vi "visualisation.vi"(8 "Joint B":dbl(knob)=5.611498737356196 scale format="%#.1f", 9 "Joint A":dbl(knob)=5.611498737356196 scale format="%#.1f", 10 "Length B":dbl(slide)=35.714285714285715 scale=10.0..80.0, 11 "Length A":dbl(slide)=70.71428571428572 scale=10.0..80.0) -> (3 "Picture":picture)   [LabVIEW 2016]
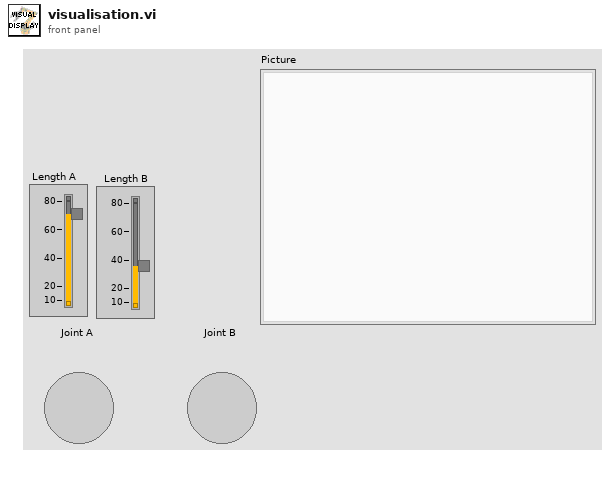
[diagram p1: front panel]
types:
  T1 = cluster{"top":dbl, "left":dbl, "height":dbl, "width":dbl}
  T2 = cluster{"Joint A":dbl, "height":dbl, "scale factor":dbl}
  T3 = cluster{"left":dbl, "top":dbl, "right":dbl, "bottom":dbl}
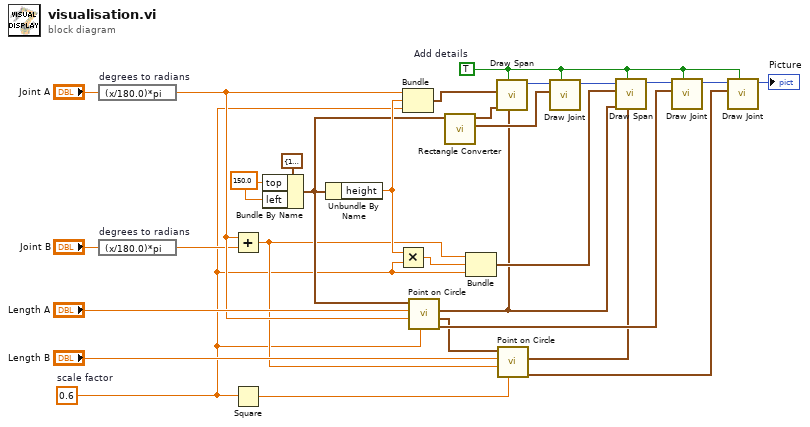
[diagram p0: block diagram]
diagram:
  w5 = TRUE  # Add details
  w2 = 0.6  # scale factor
  w1 = 150.0
  n1 = expression code="(x/180.0)*pi" "degrees to radians"("Joint A") -> (w18:dbl)
  n2 = expression code="(x/180.0)*pi" "degrees to radians"("Joint B") -> (w16:dbl)
  n3 = Add(x=w18, y=w16) -> (x+y=w4:dbl)
  n4 = Square(x=w2) -> (x^2=w13:dbl)
  n5 = Bundle By Name(cluster=T1 {"top"=120.0, "left"=70.0, "height"=32.0, "width"=32.0} ("Circle"), "top"=w1, "left"=w1) -> (w15:T1)
  n6 = Unbundle By Name(w15) -> ("height"=w26:dbl)
  n7 = Multiply(x=w26, y=w2) -> (x*y=w29:dbl)
  n8 = Bundle("Joint A"=w18, "height"=w26, "scale factor"=w2) -> (w27:T2)  [unwired: 1 in]
  n9 = call "Point on Circle.vi"("Scale Factor"=w2, "Angle"=w18, "Radius"="Length A", "Rect In"=w15) -> ("Scaled Rect Out"=w10:T3, "Rect Out"=w9:T3, "scaled point"=w11:cluster{"x":dbl, "y":dbl})  [unwired: 4 in, 1 out]
  n10 = call "Rectangle Converter.vi"("Rect"=w15) -> ("Rect Out"=w23:T3, "Center"=w14:cluster{"x":dbl, "y":dbl})  [unwired: 9 in]
  n11 = Bundle(w4, w29, "scale factor"=w2) -> (w28:cluster{dbl, dbl, "scale factor":dbl})  [unwired: 1 in]
  n12 = call "Draw Span.vi"("Center 2"=w11, "Enhance Style"=w5, "Center 1"=w14, "Circle Spec"=w27) -> ("Picture Out"=w24:picture)  [unwired: 7 in]
  n13 = call "Point on Circle.vi"("Scale Factor"=w13, "Angle"=w4, "Radius"="Length B", "Rect In"=w9) -> ("Scaled Rect Out"=w12:T3, "scaled point"=w8:cluster{"x":dbl, "y":dbl})  [unwired: 4 in, 2 out]
  n14 = call "Draw Joint.vi"("Enhance Style"=w5, "Rectangle"=w23, "Picture In"=w24) -> ("Picture Out"=w7:picture)  [unwired: 8 in]
  n15 = call "Draw Span.vi"("Center 2"=w8, "Enhance Style"=w5, "Center 1"=w11, "Circle Spec"=w28, "Picture In"=w7) -> ("Picture Out"=w25:picture)  [unwired: 6 in]
  n16 = call "Draw Joint.vi"("Enhance Style"=w5, "Rectangle"=w10, "Picture In"=w25) -> ("Picture Out"=w6:picture)  [unwired: 8 in]
  n17 = call "Draw Joint.vi"("Enhance Style"=w5, "Rectangle"=w12, "Picture In"=w6) -> ("Picture Out"=→"Picture":picture)  [unwired: 8 in]
